vi "Implementation Error.vi"(8 "error in (no error)":errorcluster) -> (0 "error out":errorcluster)   [LabVIEW 2014, in "BaseClasses.lvlib" / "BaseObject.lvclass"]
uses:
  BaseObject.lvclass
  <vilib>/Utility/error.llb/Error Cluster From Error Code.vi
  <vilib>/ErrorRing/Error Ring.xnode
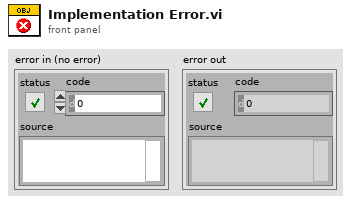
[diagram p1: front panel]
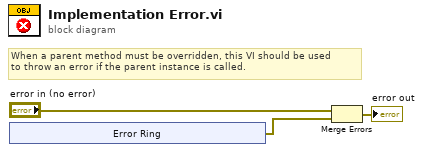
[diagram p0: block diagram]
diagram:
  # "When a parent method must be overridden, this VI should be used\nto throw an error if the parent instance is called."
  n1 = xnode "Error Ring"() -> ("error out"=w1:errorcluster)
  n2 = Merge Errors("error in (no error)", w1) -> (→"error out":errorcluster)
